vi "20181120_sin_wave.vi"() -> ()   [LabVIEW 2017]
panel:
  in  "cos_hz":dbl
  in  "sin_hz":dbl
  in  "cos":dbl
  in  "sin":dbl
  out "Waveform Chart":cluster{i32, dbl}(graph)
  in  "stop":bool
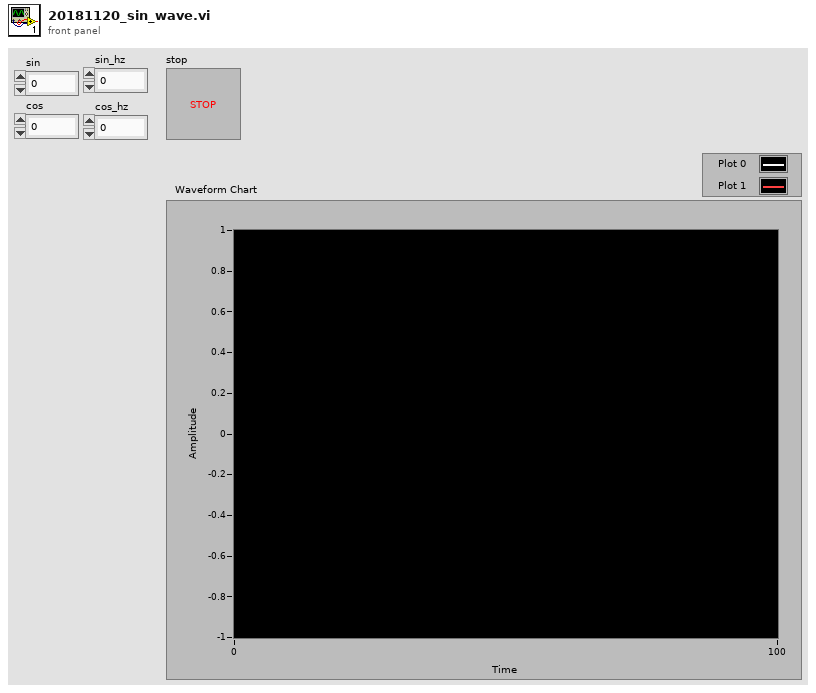
[diagram p1: front panel]
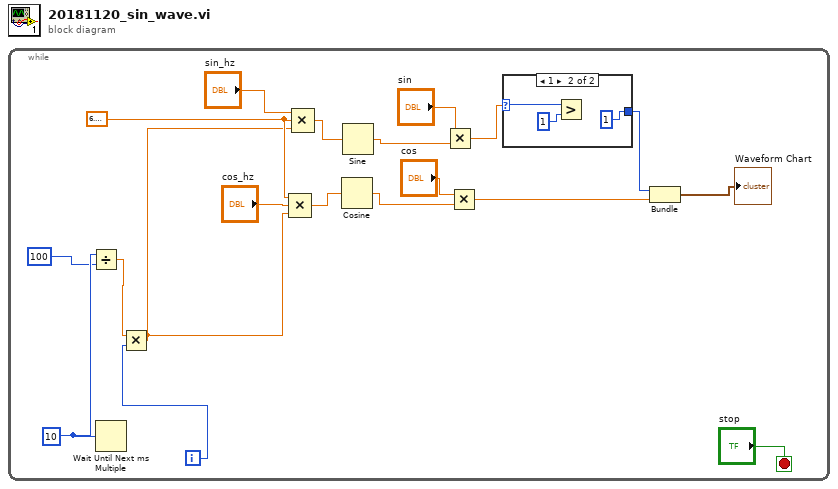
[diagram p0: block diagram]
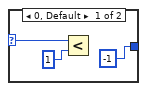
[diagram p2: hidden frame]
diagram:
  n1 = while {
    i -> [w12]
    stop <- "stop" stop-if-true
    w8 = 6.283185307179586
    w6 = 10
    n2 = Divide(x=w6, y=100) -> (x/y=w11:dbl)
    n3 = Wait Until Next ms Multiple(millisecond multiple=w6) -> ()  [unwired: 1 out]
    n4 = Multiply(x=w11, y=w12) -> (x*y=w4:dbl)
    n5 = Compound Arithmetic op=MULTIPLY(w8, "cos_hz", w4) -> (w7:dbl)
    n6 = Compound Arithmetic op=MULTIPLY("sin_hz", w8, w4) -> (w10:dbl)
    n7 = Cosine(x=w7) -> (cos(x)=w15:dbl)
    n8 = Sine(x=w10) -> (sin(x)=w17:dbl)
    n9 = Multiply(x="sin", y=w17) -> (x*y=w3:dbl)
    n10 = Multiply(x="cos", y=w15) -> (x*y=w1:dbl)
    n11 = case shown="1" w3 {
      selector: w3 -> [w21 w24]
      tunnel: [-1 1] -> w2
      frame 0, Default {
        n12 = Less?(x=w21, y=1) -> ()  [unwired: 1 out]
      }
      frame 1 {
        n13 = Greater?(x=w24, y=1) -> ()  [unwired: 1 out]
      }
    }
    n14 = Bundle(w2, w1) -> (→"Waveform Chart":cluster{i32, dbl})  [unwired: 1 in]
  }
